vi "TX Message.vi"(8 "error in (no error)":errorcluster, 10 "variant":variant, 11 "PID in":refnum<class "PID.lvclass">) -> (0 "error out":errorcluster, 3 "PID out":refnum<class "PID.lvclass">)   [LabVIEW 2011, in "PID.lvclass"]
uses:
  PID.lvclass
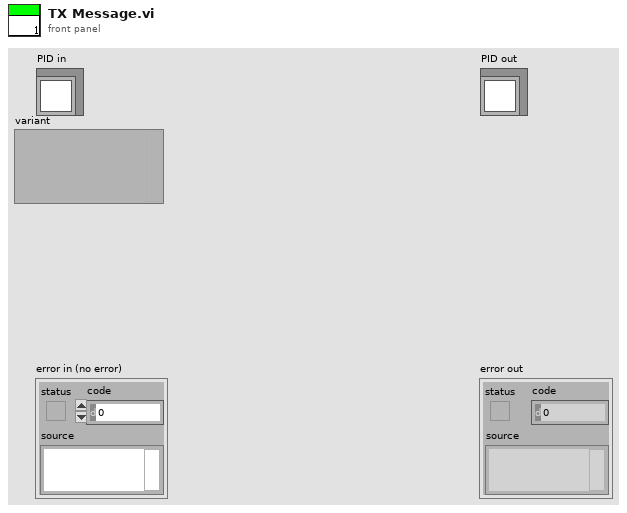
[diagram p1: front panel]
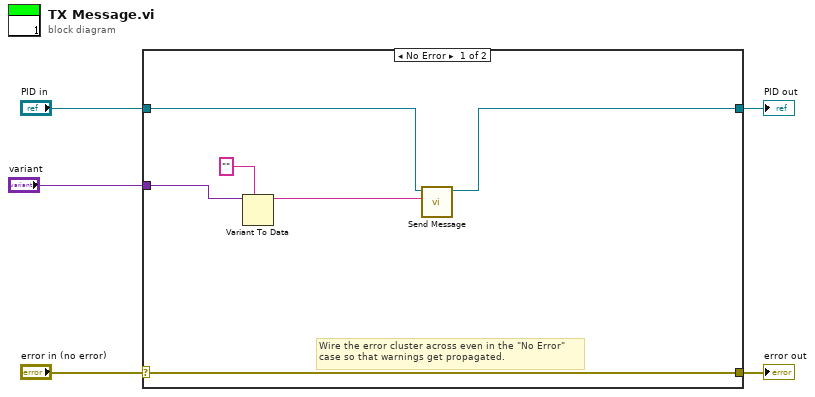
[diagram p0: block diagram]
diagram:
  n1 = case shown="No Error" "error in (no error)" {
    selector: "error in (no error)" -> [w11 w13]
    tunnel: [w11 w13] -> w4
    tunnel: [w9 w12] -> w2
    tunnel: "PID in" -> [w10 w12]
    tunnel: "variant" -> [w8 _]
    frame No Error {
      # "Wire the error cluster across even in the \"No Error\"\ncase so that warnings get propagated."
      n2 = Variant To Data(type="" ("data"), Variant=w8) -> (data=w7:string)  [unwired: 1 in, 1 out]
      n3 = call "Send Message.vi"("TX Message"=w7, "PID in"=w10) -> ("PID out"=w9:refnum<class "PID.lvclass">)  [unwired: 8 in, 1 out]
    }
    frame Error {
    }
  }
  "error out" <- w4
  "PID out" <- w2
